vi "symmetry_transform_to_marginal_evenodd_internal.vi"(4 "ROI (x,y,w,h)":i32[](array[numeric]), 5 "margin":i32=15, 6 "Transform Columns?":bool, 7 "LineWidth(Pixels)":i32, 8 "Pixel Pointer":u64 format="%.0x") -> (1 "Marginal (halfpixels)":sgl[](array[numeric]), 2 "Marginal":sgl[](array[numeric]), 3 "Pixel Pointer out":u64 format="%.0x")   [LabVIEW 2010]
panel:
  out "Marginal 2":cluster{sgl[], "xMarginal":sgl[]}[](graph)
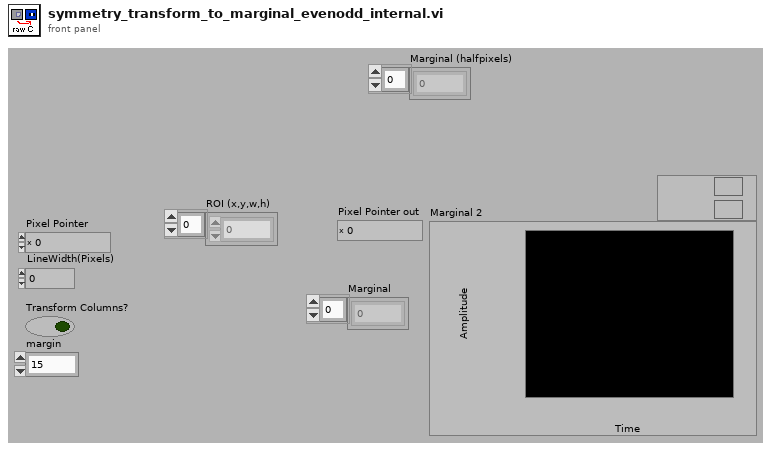
[diagram p1: front panel]
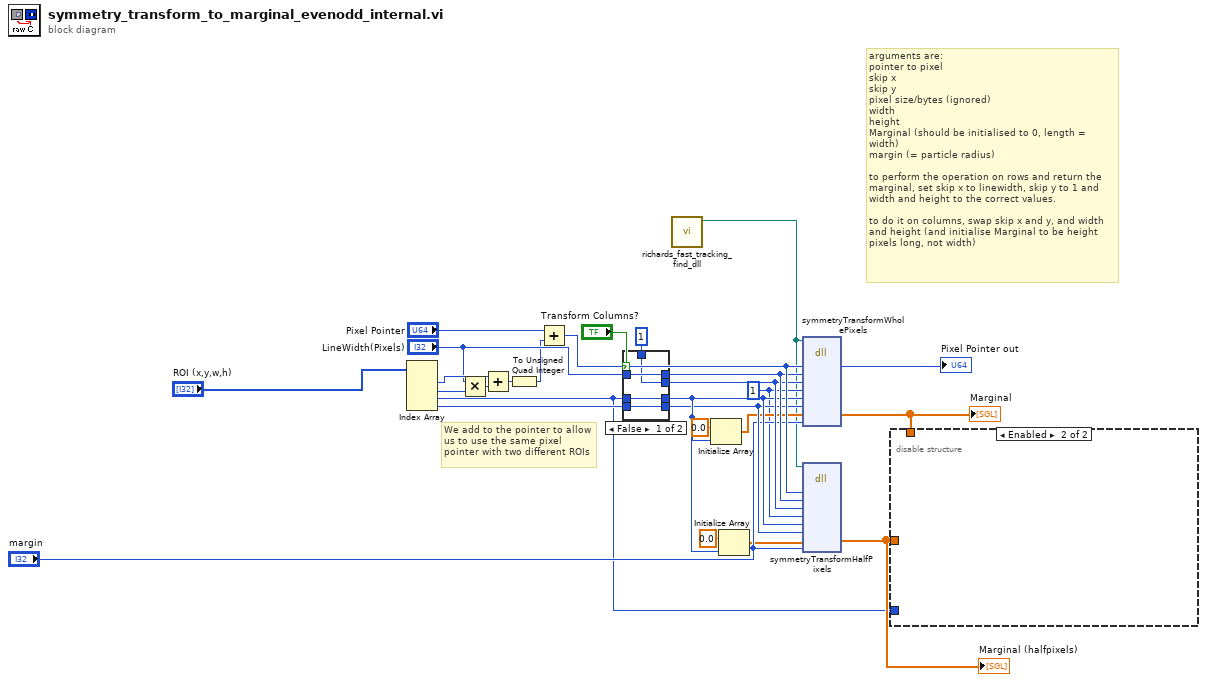
[diagram p0: block diagram]
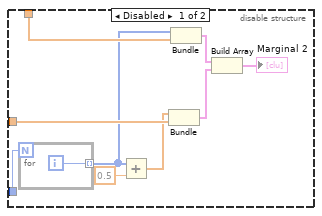
[diagram p2: hidden frame]
diagram:
  w4 = 1 ("LineWidth(Pixels)")
  # "We add to the pointer to allow us to use the same pixel pointer with two different ROIs"
  # "arguments are:\npointer to pixel\nskip x \nskip y\npixel size/bytes (ignored)\nwidth\nheight\nMarginal (should be initialised to 0, length = width)\nmargin (= particle radius)\n\nto perform the operation on rows and return the marginal, set skip x to linewidth, skip y to 1 and width and height to the correct values.\n\nto do it on columns, swap skip x and y, and width and height (and initialise Marginal to be height pixels long, not width)"
  n1 = Index Array(array="ROI (x,y,w,h)") -> (element #1=w20:i32, element #2=w22:i32, element #3=w7:i32, element #4=w25:i32)  [unwired: 4 in]
  n2 = Multiply(x="LineWidth(Pixels)", y=w22) -> (x*y=w21:i32)
  n3 = Add(x=w20, y=w21) -> (x+y=w18:i32)
  n4 = To Unsigned Quad Integer(1:w18) -> (0:w17:u64)
  n5 = Add(x="Pixel Pointer", y=w17) -> (x+y=w16:u64)
  n6 = case shown="False" "Transform Columns?" {
    tunnel: [w31 w35] -> w15
    tunnel: 1 ("LineWidth(Pixels)") -> [w30 w35]
    tunnel: [w30 w34] -> w14
    tunnel: "LineWidth(Pixels)" -> [w31 w34]
    tunnel: [w29 w32] -> w13
    tunnel: [w28 w33] -> w12
    tunnel: w7 -> [w29 w33]
    tunnel: w25 -> [w28 w32]
    frame False {
    }
    frame True {
    }
  }
  n7 = call "richards_fast_tracking_find_dll.vi"() -> ("appended path"=w1:path)  [unwired: 11 in]
  n8 = Initialize Array(sgl 0.0 ("element"), w13) -> (w5:sgl[])
  n9 = Initialize Array(sgl 0.0 ("element"), w13) -> (w2:sgl[])
  n10 = dll-call lib="C:/Users/alinnenberger/Desktop/Cube/red_tweezers_1_4_rc0/RichardFastTracking/symmetrytransform32.dll" fn="symmetryTransformWholePixels"(path in=w1, "pixelPointer"=w16, "skipx"=w15, "skipy"=w14, "pixelSizeInBytes"=w4, "width"=w13, "height"=w12, "xMarginal"=w5, "radius"="margin") -> ("pixelPointer"=→"Pixel Pointer out":u64, "xMarginal"=w9:sgl[])  [unwired: 9 in, 2 out]
  "Marginal" <- w9
  n11 = dll-call lib="C:/Users/alinnenberger/Desktop/Cube/red_tweezers_1_4_rc0/RichardFastTracking/symmetrytransform32.dll" fn="symmetryTransformHalfPixels"(path in=w1, "pixelPointer"=w16, "skipx"=w15, "skipy"=w14, "pixelSizeInBytes"=w4, "width"=w13, "height"=w12, "xMarginal"=w2, "radius"="margin") -> ("xMarginal"=w8:sgl[])  [unwired: 10 in, 2 out]
  "Marginal (halfpixels)" <- w8
  n12 = disable-structure shown="Enabled" {
    disable-tunnel: w9 -> [w44 _]
    disable-tunnel: w8 -> [w40 _]
    disable-tunnel: w7 -> [w36 _]
    frame Disabled {
      n13 = for {
        N: w36 -> [_]
        tunnel: [w45] -> w37 mode=indexing
        i -> [w45]
      }
      n14 = Add(x=w37, y=sgl 0.5) -> (x+y=w38:sgl[])
      n15 = Bundle(w38, "xMarginal"=w40) -> (w42:cluster{sgl[], "xMarginal":sgl[]})  [unwired: 1 in]
      n16 = Bundle(w37, "xMarginal"=w44) -> (w43:cluster{i32[], "xMarginal":sgl[]})  [unwired: 1 in]
      n17 = Build Array(w43, w42) -> (→"Marginal 2":cluster{sgl[], "xMarginal":sgl[]}[])
    }
    frame Enabled {
    }
  }
